vi "GM-UV-PAM.vi"() -> ()   [LabVIEW 2017]
uses:
  AlazarTech/ATS-VI/6.3.0/ATS_ctl/ATS_DMA_Channel.ctl
  <vilib>/userdefined/High Color/nirio_resource_hc.ctl
  <vilib>/FPGAPlugInAG/myRIO-1900/niLvFpga_Open_myRIO-1900.vi
  <vilib>/FPGAPlugInAG/myRIO-1900/niLvFpga_Reset_myRIO-1900.vi
  <vilib>/rvi/interface/common/niFpgaWaitOnOcc.vi
  <vilib>/Utility/error.llb/Error Cluster From Error Code.vi
  <vilib>/rvi/errors/niLvFpgaAdjustHostInterfaceError.vi
  <vilib>/FPGAPlugInAG/myRIO-1900/niLvFpga_Run_myRIO-1900.vi
  <vilib>/FPGAPlugInAG/myRIO-1900/niLvFpga_Close_myRIO-1900.vi
  <vilib>/rvi/interface/nirviOpenFPGA/nirviOpenFPGA.xnode
  FPGA Bitfiles/singlechannelMEM_FPGATarget2_MEMSMyRIO(FPGA)_jCEcXuE4l5k.lvbitx
  MEMS_MyRIO(FPGA).vi
  <vilib>/rvi/interface/nirviMethod/nirviMethod.xnode
  <vilib>/rvi/interface/nirviReadWriteControl/nirviReadWriteControl.xnode
  <vilib>/rvi/interface/nirviCloseFPGA/nirviCloseFPGA.xnode
  <vilib>/Analysis/NI_AALPro.lvlib
  <vilib>/rvi/errors/niLvFpgaMergeErrorWithErrorCode.vi
  NiFpgaLv.dll
  <vilib>/FPGAPlugInAG/myRIO-1900/niLvFpga_ConfigureFifo_myRIO-1900.vi
  <vilib>/FPGAPlugInAG/myRIO-1900/niLvFpga_WriteFifo_myRIO-1900.vi
panel:
  out "s? t:f":u16[](array[numeric])
  out "Pulses":u8[](array[numeric])
  out "Pulsesb":u8[](array[numeric])
  out "Timesperdx":i16
  in  "Savemap":bool
  in  "Calc MAP":bool
  in  "3D scan #":dbl=80.0
  out "B-scan #":u32=100
  in  "B-scan Rate":dbl=100.0 min=0.1 max=1000.0 step=0.1 format="%#_4g"
  in  "En":bool=TRUE
  in  "Mode":enum32{"Continuous", "Discrete"}(radio)
  in  "Step Size":dbl=16.0
  in  "Range (V) 2":sgl=2.0 format="%0.2f"
  in  "Offset(V)":dbl
  in  "Mirror PAM":enum32{"Main", "Others"}(tab)
  out "B-Scan 2":u16[][](graph)
  in  "pd delay":i16
  out "Laser/xn/dx should be an integer and not 1":string
  in  "Big_data":bool=TRUE
  in  "Zdiv":i8=2
  out "String 2":string="better<2^32"
  out "String":string="better<2000"
  out "Motorfreq_hz= Laserfre*dy/GMnum":dbl
  out "Stop_dispaly":bool
  in  "catbscan":i16=2
  in  "Laser Rep Rate":u32=10000 max=300000
  in  "Channel":T1
  in  "file path":path=path "G:/LXF/UV-PAM/test/test.dat"
  out "B-scan saved":i32=1600
  out "B-Scan":u16[][](graph)
  in  "Offset (V)":dbl format="%0.3f"
  in  "Range (V)":dbl=0.015 format="%0.3f"
  in  "Phase0(deg)":dbl format="%0.2f"
  in  "Trig. Delay (us)":sgl=4.3
  in  "Pt per A-line":i32=256
  in  "Rate":enum16{"500M", "250M", "125M"}(ring)
  in  "showmap":bool=TRUE
  in  "A/B-line show":bool=TRUE
  out "Alines":i32=320
  in  "Ele_Ini_Dir":bool=TRUE caption="Motor"
  out "Laser fired":i32=512000
  in  "zdir":bool
  in  "dy":i32=2 min=1 max=4
  in  "yn":i32=1000
  in  "kz":dbl=1.0
  in  "dx":i32=128
  in  "xEn":bool=TRUE
  in  "GMnum":i16=10
  in  "yEn":bool=TRUE
  in  "stop 2":bool
  in  "xn":i32=1000
  out "Waveform Graph":u16[][](graph)
  in  "ChA_Range":u32(ring)=5 items=["40 mV"=2, "100 mV"=5, "200 mV"=6, "400 mV"=7, "1 V"=10, "2 V"=11, "4 V"=12]
  in  "Triger Source":T2(ring)=enum."External"
  in  "Range Ch2":u32(ring)=3 items=["40mV", "100mV", "200mV", "400mV", "1 V", "2 V", "4 V"]
  in  "Trig Slope":enum32{"Positive", "Negative"}(ring)
  in  "Trig Level":u32=144
  out "C-Scan Ticks":dbl=300000.0
  out "Ch1 Pt":i32=384000
  out "DAQ Trig #":i32=3000
  out "Aline Stop #":i32=24000000
  out "DataQueue":refnum<queue>
  in  "signal type":T3(ring)=enum."triangle"
  out "Galvo Mirror Traj":i16[](graph)=[0, 0, 0, 1, 1, 1, 1, 2, 2, 2, 2, 2, 3, 3, 3, 3, 3, 4, 4, 4, 4, 5, 5, 5, 5, 5, 6, 6, 6, 6, 6, 7, 7, 7, 7, 7, 8, 8, 8, 8, 9, 9, 9, 9, 9, 10, 10, 10, 10, 10, 11, 11, 11, 11, 12, 12, 12, 12, 12, 13, 13, 13, 13, 13, 14, 14, 14, 14, 15, 15, 15, 15, 15, 16, 16, 16, 16, 16, 17, 17, 17, 17, 17, 18, 18, 18, 18, 19, 19, 19, 19, 19, 20, 20, 20, 20, 20, 21, 21, 21, 21, 21, 22, 22, 22, 22, 23, 23, 23, 23, 23, 24, 24, 24, 24, 24, 25, 25, 25, 25, 25, 26, 26, 26, 26, 27, 27, 27, 27, 27, 28, 28, 28, 28, 28, 29, 29, 29, 29, 29, 30, 30, 30, 30, 30, 31, 31, 31, 31, 31, 32, 32, 32, 32, 32, 33, 33, 33, 33, 33, 34, 34, 34, 34, 34, 35, 35, 35, 35, 35, 36, 36, 36, 36, 36, 37, 37, 37, 37, 37, 38, 38, 38, 38, 38, 39, 39, 39, 39, 39, 40, 40, 40, 40, 40, 41, 41, 41, 41, 41, 42, 42, 42, 42, 42, 43, 43, 43, 43, 43, 44, 44, 44, 44, 44, 45, 45, 45, 45, 45, 46, 46, 46, 46, 46, 46, 47, 47, 47, 47, 47, 48, 48, 48, 48, 48, 49, 49, 49, 49, 49, 50, 50, 50, 50, 50, 50, 51, 51, 51, 51, 51, 52, 52, 52, 52, 52, 52, 53, 53, 53, 53, 53, 54, 54, 54, 54, 54, 55, 55, 55, 55, 55, 55, 56, 56, 56, 56, 56, 56, 57, 57, 57, 57, 57, 58, 58, 58, 58, 58, 58, 59, 59, 59, 59, 59, 59, 60, 60, 60, 60, 60, 61, 61, 61, 61, 61, 61, 62, 62, 62, 62, 62, 62, 63, 63, 63, 63, 63, 63, 64, 64, 64, 64, 64, 64, 65, 65, 65, 65, 65, 65, 66, 66, 66, 66, 66, 66, 67, 67, 67, 67, 67, 67, 68, 68, 68, 68, 68, 68, 69, 69, 69, 69, 69, 69, 69, 70, 70, 70, 70, 70, 70, 71, 71, 71, 71, 71, 71, 71, 72, 72, 72, 72, 72, 72, 73, 73, 73, 73, 73, 73, 73, 74, 74, 74, 74, 74, 74, 74, 75, 75, 75, 75, 75, 75, 76, 76, 76, 76, 76, 76, 76, 77, 77, 77, 77, 77, 77, 77, 78, 78, 78, 78, 78, 78, 78, 78, 79, 79, 79, 79, 79, 79, 79, 80, 80, 80, 80, 80, 80, 80, 81, 81, 81, 81, 81, 81, 81, 81, 82, 82, 82, 82, 82, 82, 82, 82, 83, 83, 83, 83, 83, 83, 83, 83, 84, 84, 84, 84, 84, 84, 84, 84, 85, 85, 85, 85, 85, 85, 85, 85, 86, 86, 86, 86, 86, 86, 86, 86, 86, 87, 87, 87, 87, 87, 87, 87, 87, 87, 88, 88, 88, 88, 88, 88, 88, 88, 88, 89, 89, 89, 89, 89, 89, 89, 89, 89, 90, 90, 90, 90, 90, 90, 90, 90, 90, 90, 91, 91, 91, 91, 91, 91, 91, 91, 91, 91, 92, 92, 92, 92, 92, 92, 92, 92, 92, 92, 92, 93, 93, 93, 93, 93, 93, 93, 93, 93, 93, 93, 94, 94, 94, 94, 94, 94, 94, 94, 94, 94, 94, 94, 95, 95, 95, 95, 95, 95, 95, 95, 95, 95, 95, 95, 96, 96, 96, 96, 96, 96, 96, 96, 96, 96, 96, 96, 96, 96, 97, 97, 97, 97, 97, 97, 97, 97, 97, 97, 97, 97, 97, 97, 98, 98, 98, 98, 98, 98, 98, 98, 98, 98, 98, 98, 98, 98, 98, 98, 99, 99, 99, 99, 99, 99, 99, 99, 99, 99, 99, 99, 99, 99, 99, 99, 99, 99, 99, 100, 100, 100, 100, 100, 100, 100, 100, 100, 100, 100, 100, 100, 100, 100, 100, 100, 100, 100, 100, 100, 101, 101, 101, 101, 101, 101, 101, 101, 101, 101, 101, 101, 101, 101, 101, 101, 101, 101, 101, 101, 101, 101, 101, 101, 101, 101, 101, 101, 101, 102, 102, 102, 102, 102, 102, 102, 102, 102, 102, 102, 102, 102, 102, 102, 102, 102, 102, 102, 102, 102, 102, 102, 102, 102, 102, 102, 102, 102, 102, 102, 102, 102, 102, 102, 102, 102, 102, 102, 102, 102, 102, 102, 102, 102, 102, 102, 102, 102, 102, 102, 102, 102, 102, 102, 102, 102, 102, 102, 102, 102, 102, 102, 102, 102, 102, 102, 102, 102, 102, 102, 102, 102, 102, 102, 102, 102, 102, 102, 102, 102, 102, 102, 102, 102, 102, 102, 102, 102, 102, 102, 102, 102, 102, 102, 102, 102, 102, 102, 102, 102, 102, 102, 102, 102, 102, 102, 102, 102, 102, 102, 102, 102, 102, 102, 102, 102, 102, 102, 102, 102, 102, 102, 102, 102, 102, 102, 101, 101, 101, 101, 101, 101, 101, 101, 101, 101, 101, 101, 101, 101, 101, 101, 101, 101, 101, 101, 101, 101, 101, 101, 101, 101, 101, 101, 101, 100, 100, 100, 100, 100, 100, 100, 100, 100, 100, 100, 100, 100, 100, 100, 100, 100, 100, 100, 100, 100, 99, 99, 99, 99, 99, 99, 99, 99, 99, 99, 99, 99, 99, 99, 99, 99, 99, 99, 99, 98, 98, 98, 98, 98, 98, 98, 98, 98, 98, 98, 98, 98, 98, 98, 98, 97, 97, 97, 97, 97, 97, 97, 97, 97, 97, 97, 97, 97, 97, 96, 96, 96, 96, 96, 96, 96, 96, 96, 96, 96, 96, 96, 96, 95, 95, 95, 95, 95, 95, 95, 95, 95, 95, 95, 95, 94, 94, 94, 94, 94, 94, 94, 94, 94, 94, 94, 94, 93, 93, 93, 93, 93, 93, 93, 93, 93, 93, 93, 92, 92, 92, 92, 92, 92, 92, 92, 92, 92, 92, 91, 91, 91, 91, 91, 91, 91, 91, 91, 91, 90, 90, 90, 90, 90, 90, 90, 90, 90, 90, 89, 89, 89, 89, 89, 89, 89, 89, 89, 88, 88, 88, 88, 88, 88, 88, 88, 88, 87, 87, 87, 87, 87, 87, 87, 87, 87, 86, 86, 86, 86, 86, 86, 86, 86, 86, 85, 85, 85, 85, 85, 85, 85, 85, 84, 84, 84, 84, 84, 84, 84, 84, 83, 83, 83, 83, 83, 83, 83, 83, 82, 82, 82, 82, 82, 82, 82, 82, 81, 81, 81, 81, 81, 81, 81, 81, 80, 80, 80, 80, 80, 80, 80, 79, 79, 79, 79, 79, 79, 79, 78, 78, 78, 78, 78, 78, 78, 78, 77, 77, 77, 77, 77, 77, 77, 76, 76, 76, 76, 76, 76, 76, 75, 75, 75, 75, 75, 75, 74, 74, 74, 74, 74, 74, 74, 73, 73, 73, 73, 73, 73, 73, 72, 72, 72, 72, 72, 72, 71, 71, 71, 71, 71, 71, 71, 70, 70, 70, 70, 70, 70, 69, 69, 69, 69, 69, 69, 69, 68, 68, 68, 68, 68, 68, 67, 67, 67, 67, 67, 67, 66, 66, 66, 66, 66, 66, 65, 65, 65, 65, 65, 65, 64, 64, 64, 64, 64, 64, 63, 63, 63, 63, 63, 63, 62, 62, 62, 62, 62, 62, 61, 61, 61, 61, 61, 61, 60, 60, 60, 60, 60, 59, 59, 59, 59, 59, 59, 58, 58, 58, 58, 58, 58, 57, 57, 57, 57, 57, 56, 56, 56, 56, 56, 56, 55, 55, 55, 55, 55, 55, 54, 54, 54, 54, 54, 53, 53, 53, 53, 53, 52, 52, 52, 52, 52, 52, 51, 51, 51, 51, 51, 50, 50, 50, 50, 50, 50, 49, 49, 49, 49, 49, 48, 48, 48, 48, 48, 47, 47, 47, 47, 47, 46, 46, 46, 46, 46, 46, 45, 45, 45, 45, 45, 44, 44, 44, 44, 44, 43, 43, 43, 43, 43, 42, 42, 42, 42, 42, 41, 41, 41, 41, 41, 40, 40, 40, 40, 40, 39, 39, 39, 39, 39, 38, 38, 38, 38, 38, 37, 37, 37, 37, 37, 36, 36, 36, 36, 36, 35, 35, 35, 35, 35, 34, 34, 34, 34, 34, 33, 33, 33, 33, 33, 32, 32, 32, 32, 32, 31, 31, 31, 31, 31, 30, 30, 30, 30, 30, 29, 29, 29, 29, 29, 28, 28, 28, 28, 28, 27, 27, 27, 27, 27, 26, 26, 26, 26, 25, 25, 25, 25, 25, 24, 24, 24, 24, 24, 23, 23, 23, 23, 23, 22, 22, 22, 22, 21, 21, 21, 21, 21, 20, 20, 20, 20, 20, 19, 19, 19, 19, 19, 18, 18, 18, 18, 17, 17, 17, 17, 17, 16, 16, 16, 16, 16, 15, 15, 15, 15, 15, 14, 14, 14, 14, 13, 13, 13, 13, 13, 12, 12, 12, 12, 12, 11, 11, 11, 11, 10, 10, 10, 10, 10, 9, 9, 9, 9, 9, 8, 8, 8, 8, 7, 7, 7, 7, 7, 6, 6, 6, 6, 6, 5, 5, 5, 5, 5, 4, 4, 4, 4, 3, 3, 3, 3, 3, 2, 2, 2, 2, 2, 1, 1, 1, 1, 0, 0, 0, 0, 0, -1, -1, -1, -1, -2, -2, -2, -2, -2, -3, -3, -3, -3, -3, -4, -4, -4, -4, -5, -5, -5, -5, -5, -6, -6, -6, -6, -6, -7, -7, -7, -7, -7, -8, -8, -8, -8, -9, -9, -9, -9, -9, -10, -10, -10, -10, -10, -11, -11, -11, -11, -12, -12, -12, -12, -12, -13, -13, -13, -13, -13, -14, -14, -14, -14, -15, -15, -15, -15, -15, -16, -16, -16, -16, -16, -17, -17, -17, -17, -17, -18, -18, -18, -18, -19, -19, -19, -19, -19, -20, -20, -20, -20, -20, -21, -21, -21, -21, -21, -22, -22, -22, -22, -23, -23, -23, -23, -23, -24, -24, -24, -24, -24, -25, -25, -25, -25, -25, -26, -26, -26, -26, -27, -27, -27, -27, -27, -28, -28, -28, -28, -28, -29, -29, -29, -29, -29, -30, -30, -30, -30, -30, -31, -31, -31, -31, -31, -32, -32, -32, -32, -32, -33, -33, -33, -33, -33, -34, -34, -34, -34, -34, -35, -35, -35, -35, -35, -36, -36, -36, -36, -36, -37, -37, -37, -37, -37, -38, -38, -38, -38, -38, -39, -39, -39, -39, -39, -40, -40, -40, -40, -40, -41, -41, -41, -41, -41, -42, -42, -42, -42, -42, -43, -43, -43, -43, -43, -44, -44, -44, -44, -44, -45, -45, -45, -45, -45, -46, -46, -46, -46, -46, -46, -47, -47, -47, -47, -47, -48, -48, -48, -48, -48, -49, -49, -49, -49, -49, -50, -50, -50, -50, -50, -50, -51, -51, -51, -51, -51, -52, -52, -52, -52, -52, -52, -53, -53, -53, -53, -53, -54, -54, -54, -54, -54, -55, -55, -55, -55, -55, -55, -56, -56, -56, -56, -56, -56, -57, -57, -57, -57, -57, -58, -58, -58, -58, -58, -58, -59, -59, -59, -59, -59, -59, -60, -60, -60, -60, -60, -61, -61, -61, -61, -61, -61, -62, -62, -62, -62, -62, -62, -63, -63, -63, -63, -63, -63, -64, -64, -64, -64, -64, -64, -65, -65, -65, -65, -65, -65, -66, -66, -66, -66, -66, -66, -67, -67, -67, -67, -67, -67, -68, -68, -68, -68, -68, -68, -69, -69, -69, -69, -69, -69, -69, -70, -70, -70, -70, -70, -70, -71, -71, -71, -71, -71, -71, -71, -72, -72, -72, -72, -72, -72, -73, -73, -73, -73, -73, -73, -73, -74, -74, -74, -74, -74, -74, -74, -75, -75, -75, -75, -75, -75, -76, -76, -76, -76, -76, -76, -76, -77, -77, -77, -77, -77, -77, -77, -78, -78, -78, -78, -78, -78, -78, -78, -79, -79, -79, -79, -79, -79, -79, -80, -80, -80, -80, -80, -80, -80, -81, -81, -81, -81, -81, -81, -81, -81, -82, -82, -82, -82, -82, -82, -82, -82, -83, -83, -83, -83, -83, -83, -83, -83, -84, -84, -84, -84, -84, -84, -84, -84, -85, -85, -85, -85, -85, -85, -85, -85, -86, -86, -86, -86, -86, -86, -86, -86, -86, -87, -87, -87, -87, -87, -87, -87, -87, -87, -88, -88, -88, -88, -88, -88, -88, -88, -88, -89, -89, -89, -89, -89, -89, -89, -89, -89, -90, -90, -90, -90, -90, -90, -90, -90, -90, -90, -91, -91, -91, -91, -91, -91, -91, -91, -91, -91, -92, -92, -92, -92, -92, -92, -92, -92, -92, -92, -92, -93, -93, -93, -93, -93, -93, -93, -93, -93, -93, -93, -94, -94, -94, -94, -94, -94, -94, -94, -94, -94, -94, -94, -95, -95, -95, -95, -95, -95, -95, -95, -95, -95, -95, -95, -96, -96, -96, -96, -96, -96, -96, -96, -96, -96, -96, -96, -96, -96, -97, -97, -97, -97, -97, -97, -97, -97, -97, -97, -97, -97, -97, -97, -98, -98, -98, -98, -98, -98, -98, -98, -98, -98, -98, -98, -98, -98, -98, -98, -99, -99, -99, -99, -99, -99, -99, -99, -99, -99, -99, -99, -99, -99, -99, -99, -99, -99, -99, -100, -100, -100, -100, -100, -100, -100, -100, -100, -100, -100, -100, -100, -100, -100, -100, -100, -100, -100, -100, -100, -101, -101, -101, -101, -101, -101, -101, -101, -101, -101, -101, -101, -101, -101, -101, -101, -101, -101, -101, -101, -101, -101, -101, -101, -101, -101, -101, -101, -101, -102, -102, -102, -102, -102, -102, -102, -102, -102, -102, -102, -102, -102, -102, -102, -102, -102, -102, -102, -102, -102, -102, -102, -102, -102, -102, -102, -102, -102, -102, -102, -102, -102, -102, -102, -102, -102, -102, -102, -102, -102, -102, -102, -102, -102, -102, -102, -102, -102, -102, -102, -102, -102, -102, -102, -102, -102, -102, -102, -102, -102, -102, -102, -102, -102, -102, -102, -102, -102, -102, -102, -102, -102, -102, -102, -102, -102, -102, -102, -102, -102, -102, -102, -102, -102, -102, -102, -102, -102, -102, -102, -102, -102, -102, -102, -102, -102, -102, -102, -102, -102, -102, -102, -102, -102, -102, -102, -102, -102, -102, -102, -102, -102, -102, -102, -102, -102, -102, -102, -102, -102, -102, -102, -102, -102, -102, -102, -101, -101, -101, -101, -101, -101, -101, -101, -101, -101, -101, -101, -101, -101, -101, -101, -101, -101, -101, -101, -101, -101, -101, -101, -101, -101, -101, -101, -101, -100, -100, -100, -100, -100, -100, -100, -100, -100, -100, -100, -100, -100, -100, -100, -100, -100, -100, -100, -100, -100, -99, -99, -99, -99, -99, -99, -99, -99, -99, -99, -99, -99, -99, -99, -99, -99, -99, -99, -99, -98, -98, -98, -98, -98, -98, -98, -98, -98, -98, -98, -98, -98, -98, -98, -98, -97, -97, -97, -97, -97, -97, -97, -97, -97, -97, -97, -97, -97, -97, -96, -96, -96, -96, -96, -96, -96, -96, -96, -96, -96, -96, -96, -96, -95, -95, -95, -95, -95, -95, -95, -95, -95, -95, -95, -95, -94, -94, -94, -94, -94, -94, -94, -94, -94, -94, -94, -94, -93, -93, -93, -93, -93, -93, -93, -93, -93, -93, -93, -92, -92, -92, -92, -92, -92, -92, -92, -92, -92, -92, -91, -91, -91, -91, -91, -91, -91, -91, -91, -91, -90, -90, -90, -90, -90, -90, -90, -90, -90, -90, -89, -89, -89, -89, -89, -89, -89, -89, -89, -88, -88, -88, -88, -88, -88, -88, -88, -88, -87, -87, -87, -87, -87, -87, -87, -87, -87, -86, -86, -86, -86, -86, -86, -86, -86, -86, -85, -85, -85, -85, -85, -85, -85, -85, -84, -84, -84, -84, -84, -84, -84, -84, -83, -83, -83, -83, -83, -83, -83, -83, -82, -82, -82, -82, -82, -82, -82, -82, -81, -81, -81, -81, -81, -81, -81, -81, -80, -80, -80, -80, -80, -80, -80, -79, -79, -79, -79, -79, -79, -79, -78, -78, -78, -78, -78, -78, -78, -78, -77, -77, -77, -77, -77, -77, -77, -76, -76, -76, -76, -76, -76, -76, -75, -75, -75, -75, -75, -75, -74, -74, -74, -74, -74, -74, -74, -73, -73, -73, -73, -73, -73, -73, -72, -72, -72, -72, -72, -72, -71, -71, -71, -71, -71, -71, -71, -70, -70, -70, -70, -70, -70, -69, -69, -69, -69, -69, -69, -69, -68, -68, -68, -68, -68, -68, -67, -67, -67, -67, -67, -67, -66, -66, -66, -66, -66, -66, -65, -65, -65, -65, -65, -65, -64, -64, -64, -64, -64, -64, -63, -63, -63, -63, -63, -63, -62, -62, -62, -62, -62, -62, -61, -61, -61, -61, -61, -61, -60, -60, -60, -60, -60, -59, -59, -59, -59, -59, -59, -58, -58, -58, -58, -58, -58, -57, -57, -57, -57, -57, -56, -56, -56, -56, -56, -56, -55, -55, -55, -55, -55, -55, -54, -54, -54, -54, -54, -53, -53, -53, -53, -53, -52, -52, -52, -52, -52, -52, -51, -51, -51, -51, -51, -50, -50, -50, -50, -50, -50, -49, -49, -49, -49, -49, -48, -48, -48, -48, -48, -47, -47, -47, -47, -47, -46, -46, -46, -46, -46, -46, -45, -45, -45, -45, -45, -44, -44, -44, -44, -44, -43, -43, -43, -43, -43, -42, -42, -42, -42, -42, -41, -41, -41, -41, -41, -40, -40, -40, -40, -40, -39, -39, -39, -39, -39, -38, -38, -38, -38, -38, -37, -37, -37, -37, -37, -36, -36, -36, -36, -36, -35, -35, -35, -35, -35, -34, -34, -34, -34, -34, -33, -33, -33, -33, -33, -32, -32, -32, -32, -32, -31, -31, -31, -31, -31, -30, -30, -30, -30, -30, -29, -29, -29, -29, -29, -28, -28, -28, -28, -28, -27, -27, -27, -27, -27, -26, -26, -26, -26, -25, -25, -25, -25, -25, -24, -24, -24, -24, -24, -23, -23, -23, -23, -23, -22, -22, -22, -22, -21, -21, -21, -21, -21, -20, -20, -20, -20, -20, -19, -19, -19, -19, -19, -18, -18, -18, -18, -17, -17, -17, -17, -17, -16, -16, -16, -16, -16, -15, -15, -15, -15, -15, -14, -14, -14, -14, -13, -13, -13, -13, -13, -12, -12, -12, -12, -12, -11, -11, -11, -11, -10, -10, -10, -10, -10, -9, -9, -9, -9, -9, -8, -8, -8, -8, -7, -7, -7, -7, -7, -6, -6, -6, -6, -6, -5, -5, -5, -5, -5, -4, -4, -4, -4, -3, -3, -3, -3, -3, -2, -2, -2, -2, -2, -1, -1, -1, -1, 0, 0]
  in  "save_rate":u32=5
  in  "DO_rate_tick":u32=2000
  in  "Laserupdateus":u32=2000
  out "Graph":u16[][](graph)
  out "Trigger pulse graph 2":digitalwaveform(graph)={"t0"=timestamp(0 s since 1904-01-01), "dt"=0.025, "Y"={"transitions"=[], "data"=array1242x4[4968 elements]}}
  in  "Dual Wave":bool=TRUE
  in  "Split":i32=28
  out "MAP":u16[][](graph)
  out "file_ref":refnum<file>
  # "Scan"
  # "Step motor"
  # "Y Mirror"
  # "Max Rep rate 310 kHz"
  # "AD"
  # "Galvo Mirror"
  # "DAQ"
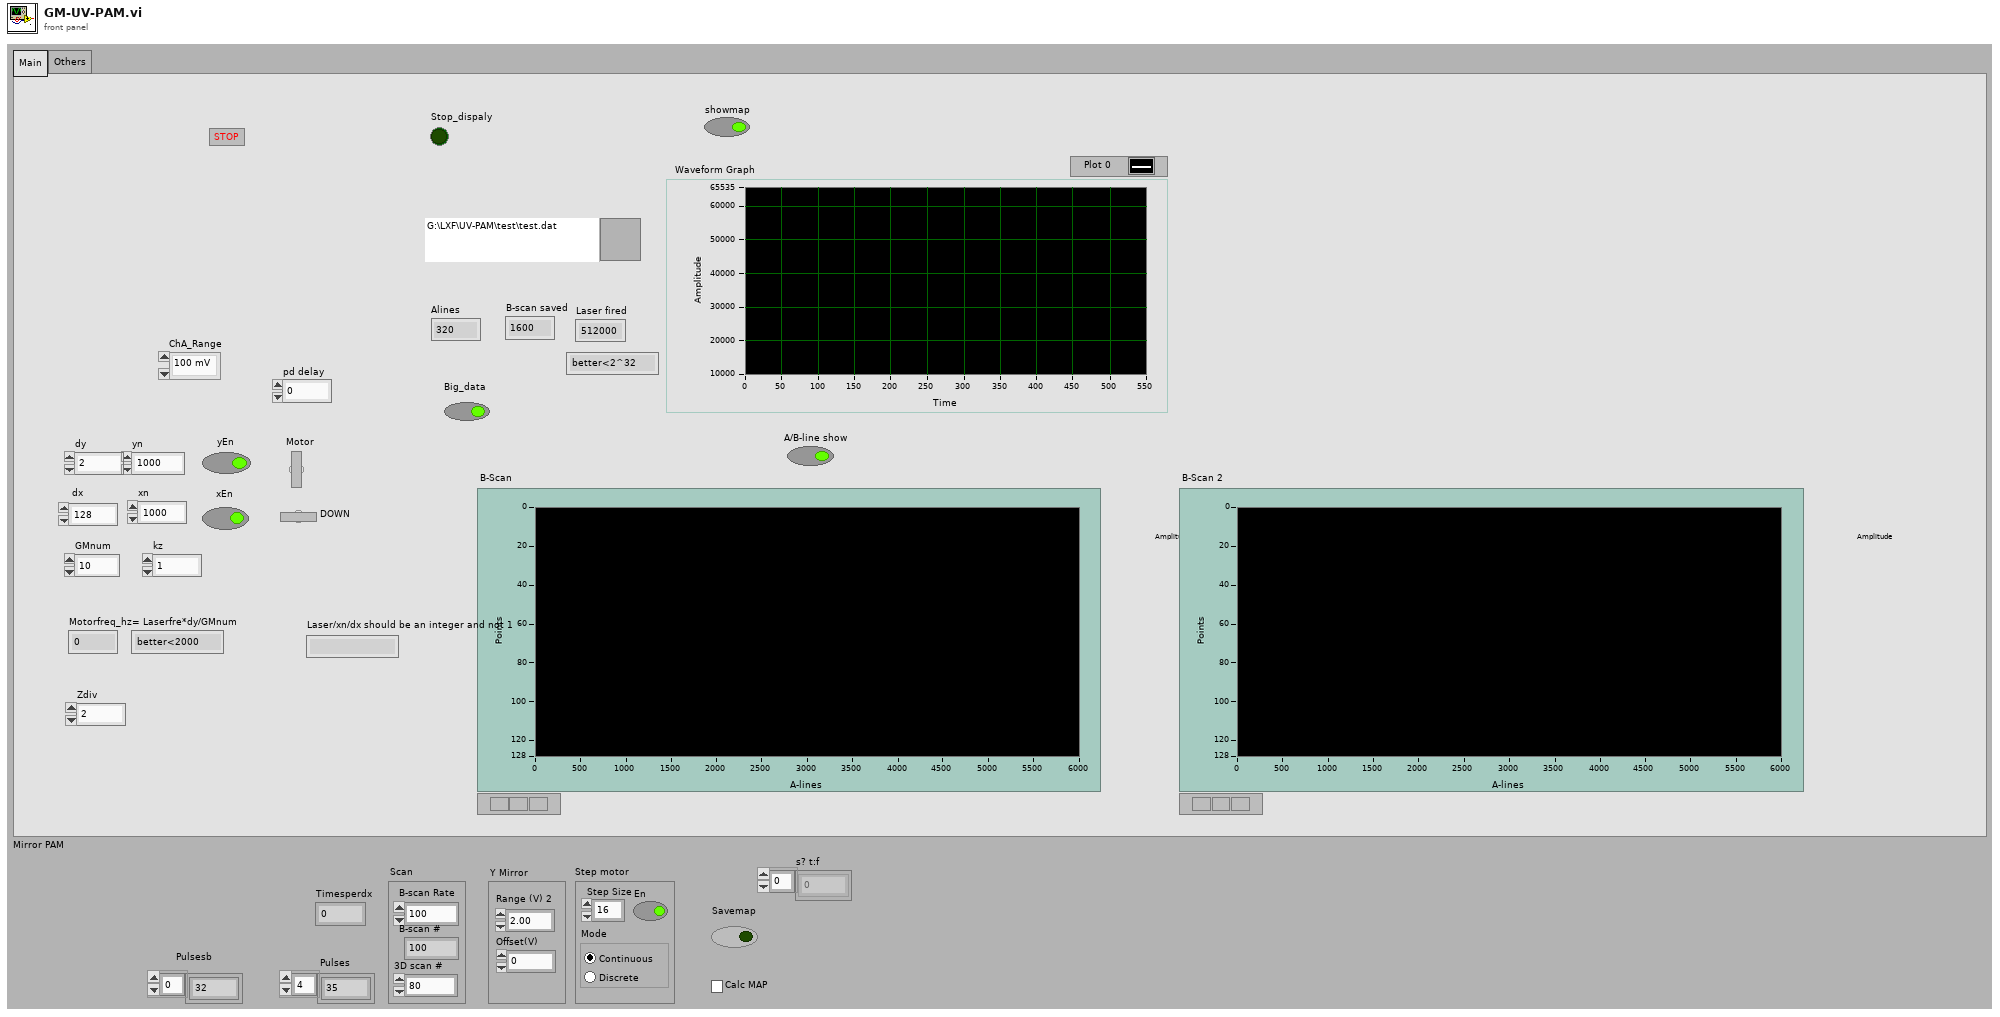
[diagram p1: front panel]
types:
  T1 = typedef "ATS_DMA_Channel.ctl" = enum16{"Channel_A", "Channel_B", "A & B"}
  T2 = enum32{"Chan_A", "Chan_B", "External", "Disable"}
  T3 = enum16{"sine", "cosine", "triangle", "square", "sawtooth", "increasing ramp", "decreasing ramp"}
  T4 = enum16{"open", "replace", "create", "open or create", "replace or create", "replace or create with confirmation"}
  T5 = enum16{"big-endian, network order", "native, host order", "little-endian"}
  T6 = typedef "nirio_resource_hc.ctl" = tag
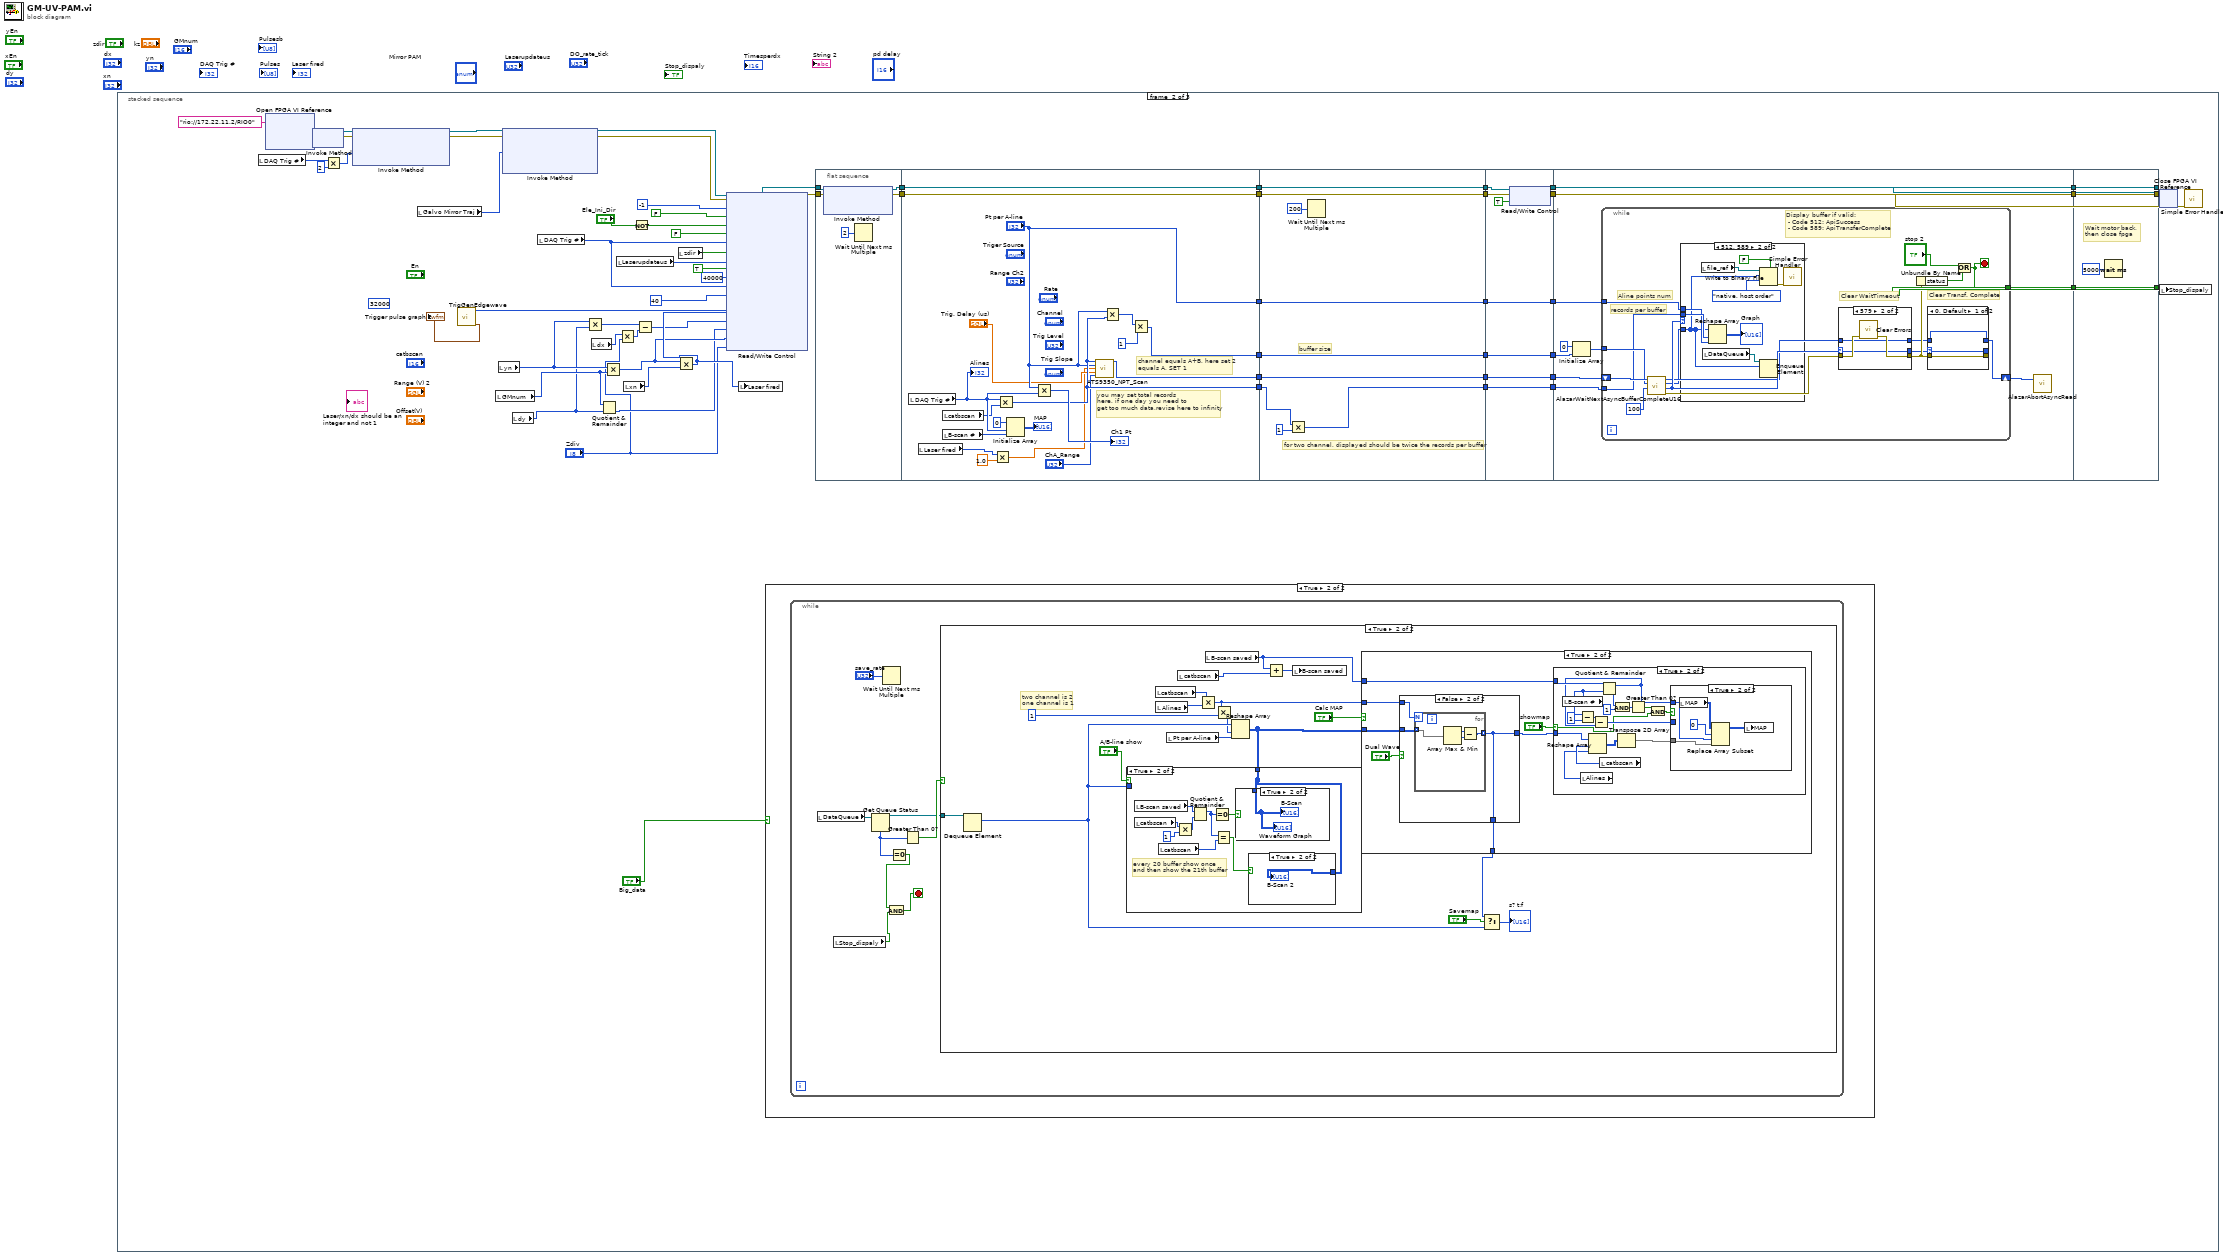
[diagram p0: block diagram]
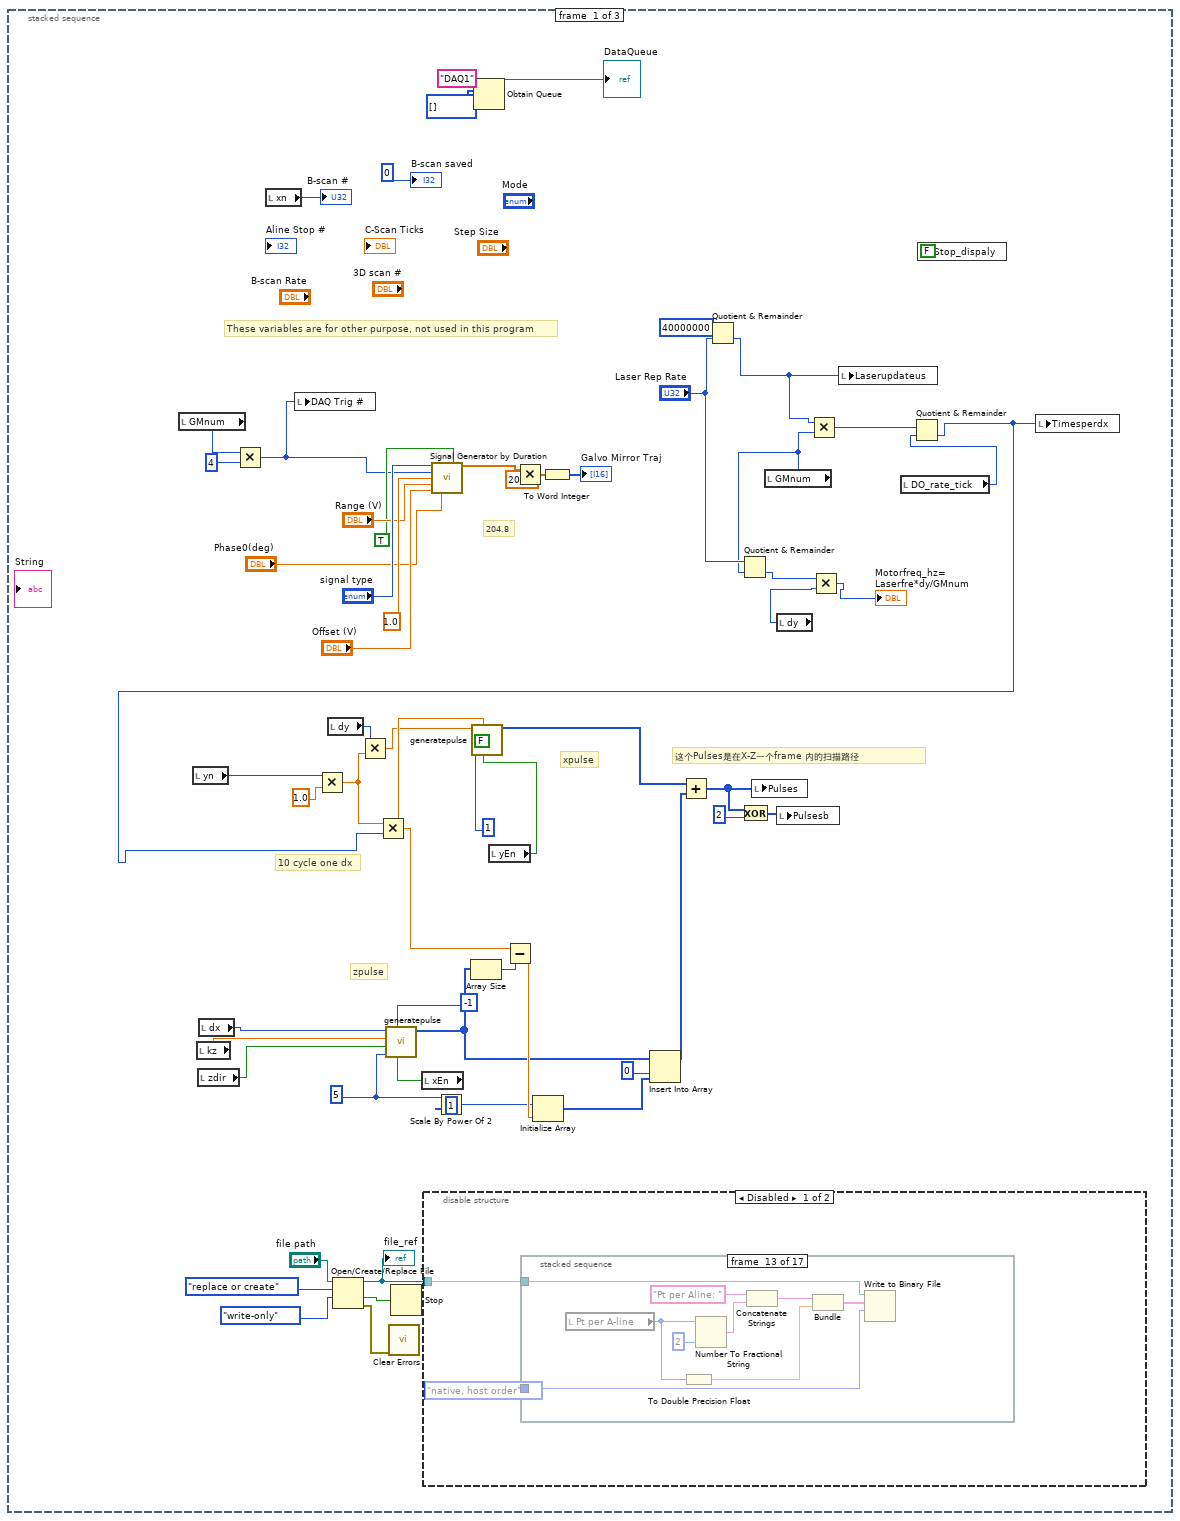
[diagram p2: hidden frame]
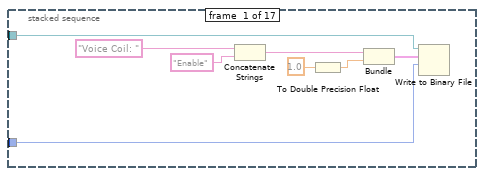
[diagram p3: hidden frame]
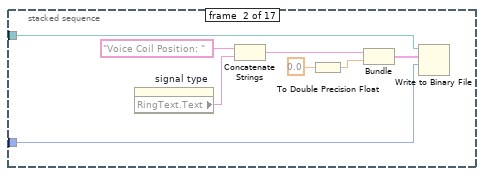
[diagram p4: hidden frame]
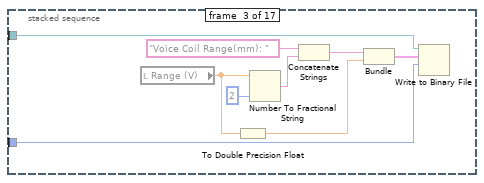
[diagram p5: hidden frame]
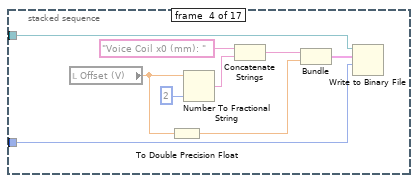
[diagram p6: hidden frame]
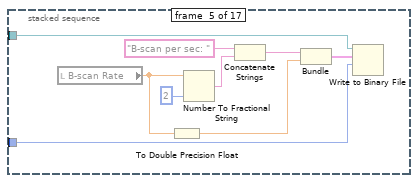
[diagram p7: hidden frame]
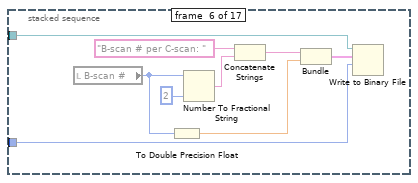
[diagram p8: hidden frame]
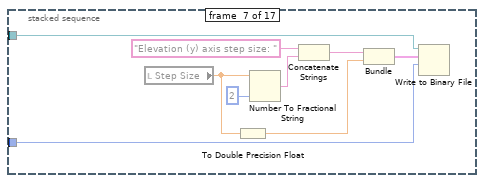
[diagram p9: hidden frame]
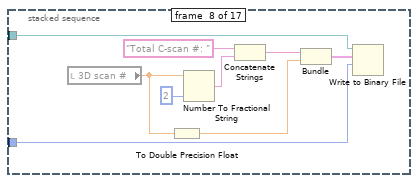
[diagram p10: hidden frame]
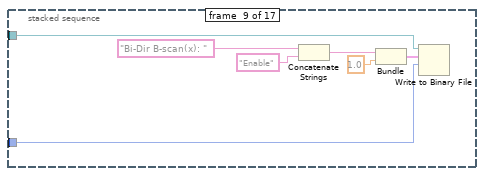
[diagram p11: hidden frame]
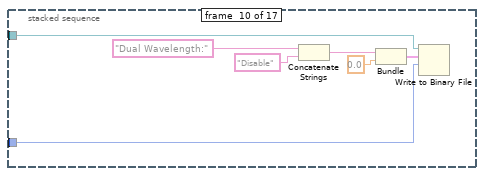
[diagram p12: hidden frame]
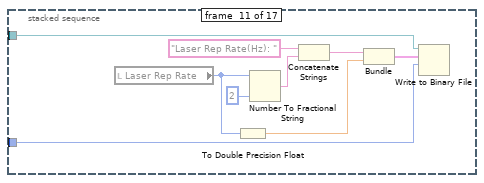
[diagram p13: hidden frame]
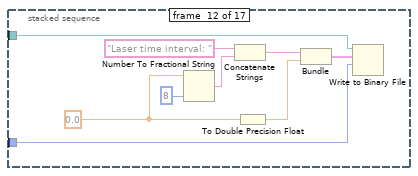
[diagram p14: hidden frame]
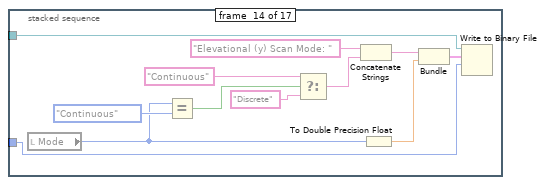
[diagram p15: hidden frame]
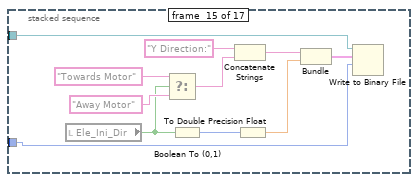
[diagram p16: hidden frame]
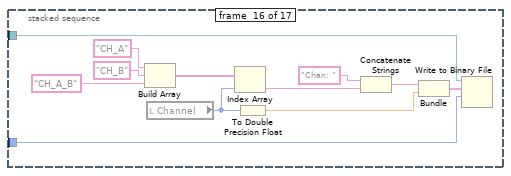
[diagram p17: hidden frame]
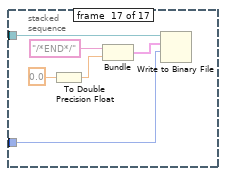
[diagram p18: hidden frame]
diagram:
  n1 = stacked-sequence {
    frame #0 {
      w18 = u8 5 ("bit")
      # "These variables are for other purpose, not used in this program"
      # "10 cycle one dx"
      # "这个Pulses是在X-Z一个frame 内的扫描路径"
      # "zpulse"
      # "xpulse"
      # "204.8"
      n2 = local read "GMnum"() -> (w16:i16)
      n3 = local read "yn"() -> (w40:i32)
      n4 = local read "kz"() -> (w24:dbl)
      n5 = local read "zdir"() -> (w23:bool)
      n6 = local read "dx"() -> (w25:i32)
      n7 = Multiply(x=w16, y=i16 4) -> (x*y=w14:i16)
      n8 = local read "xn"() -> (→"B-scan #":i32)
      n9 = local write "DAQ Trig #"(w14) -> ()
      n10 = Multiply(x=w40, y=1.0) -> (x*y=w42:dbl)
      n11 = local read "dy"() -> (w41:i32)
      n12 = Open/Create/Replace File(file path (use dialog)="file path", operation (0:open)=T4."replace or create", access (0:read/write)=enum16{"read/write", "read-only", "write-only"}."write-only") -> (refnum out=w48:refnum<file>, cancelled=w47:bool, error out=w46:errorcluster)  [unwired: 1 in, 2 out]
      "file_ref" <- w48
      n13 = Multiply(x=w41, y=w42) -> (x*y=w30:dbl)
      n14 = call <vilib>:"Clear Errors.vi"("error in (no error)"=w46) -> ()  [unwired: 5 in, 2 out]
      n15 = Stop(stop? (T)=w47) -> ()
      n16 = local read "xEn"() -> (w22:bool)
      n17 = call "generatepulse.vi"("en"=w22, "samples"=-1, "bit"=w18, "dir"=w23, "kx"=w24, "xn"=w25) -> ("pulsetrain"=w21:u8[])  [unwired: 5 in]
      n18 = disable-structure shown="Disabled" {
        disable-tunnel: w48 -> [w63 _]
        frame Disabled {
          n19 = stacked-sequence {
            tunnel: w63 -> [w71 w80 w89 w98 w104 w112 w123 w131 w141 w148 w154 w163 w171 w184 w194 w209 w215]
            tunnel: T5."native, host order" ("byte order (0:big-endian, network order)") -> [w72 w79 w88 w97 w103 w113 w122 w130 w140 w147 w153 w162 w172 w183 w193 w208 w216]
            frame #0 {
              n20 = Concatenate Strings("Voice Coil: " ("string"), "Enable") -> (w68:string)
              n21 = To Double Precision Float(number=1.0) -> (double precision float=w69:dbl)
              n22 = Bundle(w68, w69) -> (w67:cluster{string, dbl})  [unwired: 1 in]
              n23 = Write to Binary File(file (use dialog)=w71, data=w67, 9:w72) -> ()  [unwired: 3 in, 3 out]
            }
            frame #1 {
              n24 = property on="signal type" class="Enum (strict)"() -> ("RingText.Text"=w78:string)  [unwired: 2 in, 2 out]
              n25 = Concatenate Strings("Voice Coil Position: " ("string"), w78) -> (w74:string)
              n26 = To Double Precision Float(number=0.0) -> (double precision float=w76:dbl)
              n27 = Bundle(w74, w76) -> (w75:cluster{string, dbl})  [unwired: 1 in]
              n28 = Write to Binary File(file (use dialog)=w80, data=w75, 9:w79) -> ()  [unwired: 2 in, 4 out]
            }
            frame #2 {
              n29 = local read "Range (V)"() -> (w81:dbl)
              n30 = To Double Precision Float(number=w81) -> (double precision float=w84:dbl)
              n31 = Number To Fractional String(number=w81, precision (6)=i16 2) -> (F-format string=w86:string)  [unwired: 2 in]
              n32 = Concatenate Strings("Voice Coil Range(mm): " ("string"), w86) -> (w82:string)
              n33 = Bundle(w82, w84) -> (w83:cluster{string, dbl})  [unwired: 1 in]
              n34 = Write to Binary File(file (use dialog)=w89, data=w83, 9:w88) -> ()  [unwired: 2 in, 4 out]
            }
            frame #3 {
              n35 = local read "Offset (V)"() -> (w90:dbl)
              n36 = To Double Precision Float(number=w90) -> (double precision float=w93:dbl)
              n37 = Number To Fractional String(number=w90, precision (6)=i16 2) -> (F-format string=w95:string)  [unwired: 2 in]
              n38 = Concatenate Strings("Voice Coil x0 (mm): " ("string"), w95) -> (w91:string)
              n39 = Bundle(w91, w93) -> (w92:cluster{string, dbl})  [unwired: 1 in]
              n40 = Write to Binary File(file (use dialog)=w98, data=w92, 9:w97) -> ()  [unwired: 2 in, 4 out]
            }
            frame #4 {
              n41 = local read "B-scan Rate"() -> (w99:dbl)
              n42 = To Double Precision Float(number=w99) -> (double precision float=w102:dbl)
              n43 = Number To Fractional String(number=w99, precision (6)=i16 2) -> (F-format string=w106:string)  [unwired: 2 in]
              n44 = Concatenate Strings("B-scan per sec: " ("string"), w106) -> (w100:string)
              n45 = Bundle(w100, w102) -> (w101:cluster{string, dbl})  [unwired: 1 in]
              n46 = Write to Binary File(file (use dialog)=w104, data=w101, 9:w103) -> ()  [unwired: 2 in, 4 out]
            }
            frame #5 {
              n47 = local read "B-scan #"() -> (w108:u32)
              n48 = To Double Precision Float(number=w108) -> (double precision float=w111:dbl)
              n49 = Number To Fractional String(number=w108, precision (6)=i16 2) -> (F-format string=w115:string)  [unwired: 2 in]
              n50 = Concatenate Strings("B-scan # per C-scan: " ("string"), w115) -> (w109:string)
              n51 = Bundle(w109, w111) -> (w110:cluster{string, dbl})  [unwired: 1 in]
              n52 = Write to Binary File(file (use dialog)=w112, data=w110, 9:w113) -> ()  [unwired: 2 in, 4 out]
            }
            frame #6 {
              n53 = local read "Step Size"() -> (w117:dbl)
              n54 = To Double Precision Float(number=w117) -> (double precision float=w120:dbl)
              n55 = Number To Fractional String(number=w117, precision (6)=i16 2) -> (F-format string=w121:string)  [unwired: 2 in]
              n56 = Concatenate Strings("Elevation (y) axis step size: " ("string"), w121) -> (w118:string)
              n57 = Bundle(w118, w120) -> (w119:cluster{string, dbl})  [unwired: 1 in]
              n58 = Write to Binary File(file (use dialog)=w123, data=w119, 9:w122) -> ()  [unwired: 2 in, 4 out]
            }
            frame #7 {
              n59 = local read "3D scan #"() -> (w126:dbl)
              n60 = To Double Precision Float(number=w126) -> (double precision float=w129:dbl)
              n61 = Number To Fractional String(number=w126, precision (6)=i16 2) -> (F-format string=w133:string)  [unwired: 2 in]
              n62 = Concatenate Strings("Total C-scan #: " ("string"), w133) -> (w127:string)
              n63 = Bundle(w127, w129) -> (w128:cluster{string, dbl})  [unwired: 1 in]
              n64 = Write to Binary File(file (use dialog)=w131, data=w128, 9:w130) -> ()  [unwired: 2 in, 4 out]
            }
            frame #8 {
              n65 = Concatenate Strings("Bi-Dir B-scan(x): " ("string"), "Enable") -> (w138:string)
              n66 = Bundle(w138, "double precision float"=1.0) -> (w137:cluster{string, "double precision float":dbl})  [unwired: 1 in]
              n67 = Write to Binary File(file (use dialog)=w141, data=w137, 9:w140) -> ()  [unwired: 2 in, 4 out]
            }
            frame #9 {
              n68 = Concatenate Strings("Dual Wavelength:" ("string"), "Disable") -> (w144:string)
              n69 = Bundle(w144, 0.0) -> (w145:cluster{string, dbl})  [unwired: 1 in]
              n70 = Write to Binary File(file (use dialog)=w148, data=w145, 9:w147) -> ()  [unwired: 2 in, 4 out]
            }
            frame #10 {
              n71 = local read "Laser Rep Rate"() -> (w149:u32)
              n72 = To Double Precision Float(number=w149) -> (double precision float=w152:dbl)
              n73 = Number To Fractional String(number=w149, precision (6)=i16 2) -> (F-format string=w156:string)  [unwired: 2 in]
              n74 = Concatenate Strings("Laser Rep Rate(Hz): " ("string"), w156) -> (w150:string)
              n75 = Bundle(w150, w152) -> (w151:cluster{string, dbl})  [unwired: 1 in]
              n76 = Write to Binary File(file (use dialog)=w154, data=w151, 9:w153) -> ()  [unwired: 2 in, 4 out]
            }
            frame #11 {
              w158 = 0.0 ("number")
              n77 = Number To Fractional String(number=w158, precision (6)=i16 8) -> (F-format string=w165:string)  [unwired: 2 in]
              n78 = Concatenate Strings("Laser time interval: " ("string"), w165) -> (w159:string)
              n79 = To Double Precision Float(number=w158) -> (double precision float=w161:dbl)
              n80 = Bundle(w159, w161) -> (w160:cluster{string, dbl})  [unwired: 1 in]
              n81 = Write to Binary File(file (use dialog)=w163, data=w160, 9:w162) -> ()  [unwired: 2 in, 4 out]
            }
            frame #12 {
              n82 = local read "Pt per A-line"() -> (w167:i32)
              n83 = To Double Precision Float(number=w167) -> (double precision float=w170:dbl)
              n84 = Number To Fractional String(number=w167, precision (6)=i16 2) -> (F-format string=w174:string)  [unwired: 2 in]
              n85 = Concatenate Strings("Pt per Aline: " ("string"), w174) -> (w168:string)
              n86 = Bundle(w168, w170) -> (w169:cluster{string, dbl})  [unwired: 1 in]
              n87 = Write to Binary File(file (use dialog)=w171, data=w169, 9:w172) -> ()  [unwired: 2 in, 4 out]
            }
            frame #13 {
              n88 = local read "Mode"() -> (w176:enum32{"Continuous", "Discrete"})
              n89 = Equal?(x=w176, y=enum32{"Continuous", "Discrete"}."Continuous" ("Elevational Mode")) -> (x = y?=w181:bool)
              n90 = Select(t="Continuous", s=w181, f="Discrete") -> (s? t:f=w185:string)
              n91 = Concatenate Strings("Elevational (y) Scan Mode: " ("string"), w185) -> (w177:string)
              n92 = To Double Precision Float(number=w176) -> (double precision float=w179:dbl)
              n93 = Bundle(w177, w179) -> (w178:cluster{string, dbl})  [unwired: 1 in]
              n94 = Write to Binary File(file (use dialog)=w184, data=w178, 9:w183) -> ()  [unwired: 2 in, 4 out]
            }
            frame #14 {
              n95 = local read "Ele_Ini_Dir"() -> (w189:bool)
              n96 = Select(t="Towards Motor", s=w189, f="Away Motor") -> (s? t:f=w195:string)
              n97 = Boolean To (0,1)(Boolean=w189) -> (0, 1=w188:i16)
              n98 = Concatenate Strings("Y Direction:" ("string"), w195) -> (w191:string)
              n99 = To Double Precision Float(number=w188) -> (double precision float=w192:dbl)
              n100 = Bundle(w191, w192) -> (w190:cluster{string, dbl})  [unwired: 1 in]
              n101 = Write to Binary File(file (use dialog)=w194, data=w190, 9:w193) -> ()  [unwired: 2 in, 4 out]
            }
            frame #15 {
              n102 = Build Array("CH_A", "CH_B", "CH_A_B") -> (w204:string[])
              n103 = local read "Channel"() -> (w199:T1)
              n104 = Index Array(array=w204, index=w199) -> (element=w203:string)
              n105 = To Double Precision Float(number=w199) -> (double precision float=w202:dbl)
              n106 = Concatenate Strings("Chan: " ("string"), w203) -> (w201:string)
              n107 = Bundle(w201, w202) -> (w200:cluster{string, dbl})  [unwired: 1 in]
              n108 = Write to Binary File(file (use dialog)=w209, data=w200, 9:w208) -> ()  [unwired: 2 in, 4 out]
            }
            frame #16 {
              n109 = To Double Precision Float(number=0.0) -> (double precision float=w212:dbl)
              n110 = Bundle("/*END*/", w212) -> (w213:cluster{string, dbl})  [unwired: 1 in]
              n111 = Write to Binary File(file (use dialog)=w215, data=w213, 9:w216) -> ()  [unwired: 2 in, 4 out]
            }
          }
        }
        frame Enabled {
        }
      }
      n112 = call <vilib>:"Signal Generator by Duration.vi"("signal type"="signal type", "reset phase"=TRUE, "# of samples"=w14, "frequency"=1.0, "amplitude"="Range (V)", "dc offset"="Offset (V)", "phase in"="Phase0(deg)") -> ("signal"=w49:dbl[])  [unwired: 5 in, 3 out]
      n113 = Scale By Power Of 2(n=w18, x=u8 1 ("bit")) -> (x*2^n=w33:u8)
      n114 = Array Size(array=w21) -> (size(s)=w34:i32)
      n115 = Obtain Queue(name (unnamed)="DAQ1", element data type=u16[] [] ("Buffer")) -> (queue out=→"DataQueue":refnum<queue>)  [unwired: 3 in, 2 out]
      n116 = local read "yEn"() -> (w28:bool)
      n117 = Multiply(x=w49, y=204.8 ("frequency")) -> (x*y=w61:dbl[])
      n118 = To Word Integer(number=w61) -> (16bit integer=→"Galvo Mirror Traj":i16[])
      n119 = Quotient & Remainder(x=40000000, y="Laser Rep Rate") -> (floor(x/y)=w10:u32)  [unwired: 1 out]
      n120 = local read "GMnum"() -> (w4:i16)
      n121 = Quotient & Remainder(x="Laser Rep Rate", y=w4) -> (floor(x/y)=w3:u32)  [unwired: 1 out]
      n122 = local read "dy"() -> (w2:i32)
      n123 = Multiply(x=w10, y=w4) -> (x*y=w9:u32)
      n124 = Multiply(x=w3, y=w2) -> (x*y=→"Motorfreq_hz= Laserfre*dy/GMnum":u32)
      n125 = local write "Laserupdateus"(w10) -> ()
      n126 = local read "DO_rate_tick"() -> (w8:u32)
      n127 = Quotient & Remainder(x=w9, y=w8) -> (floor(x/y)=w7:u32)  [unwired: 1 out]
      n128 = Multiply(x=w42, y=w7) -> (x*y=w31:dbl)
      n129 = call "generatepulse.vi"("en"=w28, "samples"=w31, "bit"=u8 1, "dir"=FALSE, "xn"=w30) -> ("pulsetrain"=w27:u8[])  [unwired: 6 in]
      n130 = Subtract(x=w31, y=w34) -> (x-y=w39:dbl)
      n131 = Initialize Array(w33, w39) -> (w35:u8[])
      n132 = Insert Into Array(array=w21, index=0, new element=w35) -> (w36:u8[])
      n133 = Add(x=w27, y=w36) -> (x+y=w37:u8[])
      n134 = Exclusive Or(1:u8 2 ("bit"), 2:w37) -> (0:w38:u8[])
      n135 = local write "Pulses"(w37) -> ()
      n136 = local write "Pulsesb"(w38) -> ()
      n137 = local write "Stop_dispaly"(FALSE ("Stop_dispaly")) -> ()
      n138 = local write "Timesperdx"(w7) -> ()
      "B-scan saved" <- 0 ("saved bscan")
    }
    frame #1 {
      (unwired) i16 32000 ("pls_V")
      n139 = local read "DAQ Trig #"() -> (w274:i32)
      n140 = xnode "Open FPGA VI Reference"("resource name"=T6 "rio://172.22.11.2/RIO0") -> ("FPGA VI Reference Out"=w280:refnum<k20>, "error out"=w281:errorcluster)  [unwired: 1 in]
      n141 = xnode "Invoke Method"("FPGA VI Reference In"=w280, "error in"=w281) -> ("FPGA VI Reference Out"=w282:refnum<k20>, "error out"=w283:errorcluster)
      n142 = Multiply(x=w274, y=2) -> (x*y=w273:i32)
      n143 = xnode "Invoke Method"("FPGA VI Reference In"=w282, "error in"=w283, "Requested Depth"=w273) -> ("FPGA VI Reference Out"=w234:refnum<k20>, "error out"=w233:errorcluster)  [unwired: 1 out]
      n144 = local read "Galvo Mirror Traj"() -> (w264:i16[])
      n145 = call "TrigGenEdgewave.vi"() -> ("Digital Waveform Graph"=→"Trigger pulse graph 2":digitalwaveform, "delays"=w241:u32[])  [unwired: 10 in]
      n146 = local read "GMnum"() -> (w229:i16)
      n147 = local read "yn"() -> (w227:i32)
      n148 = xnode "Invoke Method"("FPGA VI Reference In"=w234, "error in"=w233, "Data"=w264) -> ("FPGA VI Reference Out"=w271:refnum<k20>, "error out"=w284:errorcluster)  [unwired: 1 in, 1 out]
      n149 = local read "dy"() -> (w226:i32)
      n150 = local read "DAQ Trig #"() -> (w244:i32)
      n151 = Multiply(x=w227, y=w226) -> (x*y=w225:i32)
      n152 = local read "dx"() -> (w219:i32)
      n153 = Quotient & Remainder(x=w229, y=w226) -> (floor(x/y)=w228:i32)  [unwired: 1 out]
      n154 = Multiply(x=w227, y=w229) -> (x*y=w230:i32)
      n155 = local read "Laserupdateus"() -> (w235:u32)
      n156 = Multiply(x=w219, y="Zdiv") -> (x*y=w220:i32)
      n157 = local read "xn"() -> (w240:i32)
      n158 = Not(x="Ele_Ini_Dir") -> (.not. x?=w265:bool)
      n159 = Subtract(x=w225, y=w220) -> (x-y=w232:i32)
      n160 = Multiply(x=w230, y=w240) -> (x*y=w237:i32)
      n161 = local read "zdir"() -> (w231:bool)
      n162 = xnode "Read/Write Control"("FPGA VI Reference In"=w271, "error in"=w284, "FIFO_Timeout"=-1, "stop 2"=FALSE ("stop"), "Ele_Ini_Dir"=w265, "start_scan"=FALSE, "VC_pt_in_fifo"=w244, "Zdir"=w231, "Laserupdateus"=w235, "LON"=TRUE, "Zmotorbackspeedticks"=u32 40000, "VC_pt_nm"=w244, "LsrCtrl"=40, "delays"=w241, "LaserNum"=w237, "Xn-dz"=w232, "Laser/xn/dx"=w228, "Stepm_pt_nm"=w230, "Zdiv"="Zdiv") -> ("FPGA VI Reference Out"=w278:refnum<k20>, "error out"=w275:errorcluster)
      n163 = local write "Laser fired"(w237) -> ()
      n164 = case shown="True" "Big_data" {
        frame False {
        }
        frame True {
          n165 = while {
            stop <- w285 stop-if-true
            n166 = local read "DataQueue"() -> (w292:refnum<queue>)
            n167 = local read "Stop_dispaly"() -> (w286:bool)
            n168 = Get Queue Status(queue=w292) -> (queue out=w290:refnum<queue>, # elements in queue=w289:i32)  [unwired: 2 in, 6 out]
            n169 = Wait Until Next ms Multiple(millisecond multiple="save_rate") -> ()  [unwired: 1 out]
            n170 = Equal To 0?(x=w289) -> (x = 0?=w287:bool)
            n171 = And(x=w287, y=w286) -> (x .and. y?=w285:bool)
            n172 = Greater Than 0?(x=w289) -> (x > 0?=w291:bool)
            n173 = case shown="True" w291 {
              tunnel: w290 -> [_ w310]
              frame False {
                n174 = Wait Until Next ms Multiple(millisecond multiple=u32 5) -> ()  [unwired: 1 out]
              }
              frame True {
                # "two channel is 2\none channel is 1"
                n175 = Dequeue Element(queue=w310) -> (element=w299:u16[])  [unwired: 2 in, 3 out]
                n176 = local read "catbscan"() -> (w307:i16)
                n177 = local read "Alines"() -> (w308:i32)
                n178 = local read "Pt per A-line"() -> (w303:i32)
                n179 = local read "catbscan"() -> (w298:i16)
                n180 = Multiply(x=w307, y=w308) -> (x*y=w296:i32)
                n181 = local read "B-scan saved"() -> (w304:i32)
                n182 = Multiply(x=w296, y=1) -> (x*y=w294:i32)
                n183 = Reshape Array(w299, w294, w303) -> (w306:u16[][])
                n184 = case shown="True" "A/B-line show" {
                  tunnel: w299 -> [_ _]
                  tunnel: w306 -> [_ w312]
                  frame False {
                  }
                  frame True {
                    # "every 20 buffer show once\nand then show the 21th buffer"
                    n185 = local read "B-scan saved"() -> (w316:i32)
                    n186 = local read "catbscan"() -> (w317:i16)
                    n187 = local read "catbscan"() -> (w311:i16)
                    n188 = Multiply(x=w317, y=1) -> (x*y=w319:i32)
                    n189 = Quotient & Remainder(x=w316, y=w319) -> (x-y*floor(x/y)=w314:i32)  [unwired: 1 out]
                    n190 = Equal To 0?(x=w314) -> (x = 0?=w315:bool)
                    n191 = Equal?(x=w314, y=w311) -> (x = y?=w313:bool)
                    n192 = case shown="True" w315 {
                      tunnel: w312 -> [_ w321]
                      frame False {
                      }
                      frame True {
                        "B-Scan" <- w321
                        "Waveform Graph" <- w321
                      }
                    }
                    n193 = case shown="True" w313 {
                      tunnel: w312 -> [_ w320]
                      frame False {
                      }
                      frame True {
                        "B-Scan 2" <- w320
                      }
                    }
                  }
                }
                n194 = Add(x=w304, y=w298) -> (x+y=w305:i32)
                n195 = local write "B-scan saved"(w305) -> ()
                n196 = case shown="True" "Calc MAP" {
                  tunnel: w296 -> [_ w329]
                  tunnel: w304 -> [_ w328]
                  tunnel: w306 -> [_ w327]
                  tunnel: [u16[] [] w325] -> w300
                  frame False {
                  }
                  frame True {
                    n197 = case shown="False" "Dual Wave" {
                      tunnel: w329 -> [w334 w347]
                      tunnel: w327 -> [w333 w346]
                      tunnel: [w331 w345] -> w325
                      tunnel: [w330 w345] -> w324
                      frame True {
                        n198 = for {
                          N: w334 -> [_]
                          tunnel: w333 -> [w341] mode=indexing
                          tunnel: [w344] -> w330 mode=indexing
                          tunnel: [w337] -> w332 mode=indexing
                          n199 = Split 1D Array(array=w341, index="Split") -> (first subarray=w335:u16[], second subarray=w336:u16[])
                          n200 = Array Max & Min(array=w336) -> (max value=w343:u16, min value=w342:u16)  [unwired: 2 out]
                          n201 = Array Max & Min(array=w335) -> (max value=w339:u16, min value=w338:u16)  [unwired: 2 out]
                          n202 = Subtract(x=w343, y=w342) -> (x-y=w344:u16)
                          n203 = Subtract(x=w339, y=w338) -> (x-y=w337:u16)
                        }
                        n204 = Interleave 1D Arrays(w330, w332) -> (w331:u16[])
                      }
                      frame False {
                        n205 = for {
                          N: w347 -> [_]
                          tunnel: w346 -> [w348] mode=indexing
                          tunnel: [w351] -> w345 mode=indexing
                          n206 = Array Max & Min(array=w348) -> (max value=w350:u16, min value=w349:u16)  [unwired: 2 out]
                          n207 = Subtract(x=w350, y=w349) -> (x-y=w351:u16)
                        }
                      }
                    }
                    n208 = case shown="True" "showmap" {
                      selector: "showmap" -> [_ w352]
                      tunnel: w328 -> [_ w368]
                      tunnel: w324 -> [_ w355]
                      frame False {
                      }
                      frame True {
                        n209 = local read "B-scan #"() -> (w361:u32)
                        n210 = Subtract(x=w361, y=1) -> (x-y=w365:u32)
                        n211 = local read "Alines"() -> (w359:i32)
                        n212 = local read "catbscan"() -> (w360:i16)
                        n213 = Reshape Array(w355, w360, w359) -> (w356:u16[][])
                        n214 = Quotient & Remainder(x=w368, y=w361) -> (x-y*floor(x/y)=w364:u32, floor(x/y)=w367:u32)
                        n215 = Subtract(x=w365, y=w364) -> (x-y=w363:u32)
                        n216 = And(x=w367, y=1) -> (x .and. y?=w362:u32)
                        n217 = Transpose 2D Array(2D array=w356) -> (transposed array=w358:u16[][])
                        n218 = Greater Than 0?(x=w362) -> (x > 0?=w354:bool)
                        n219 = And(x=w354, y=w352) -> (x .and. y?=w353:bool)
                        n220 = case shown="True" w353 {
                          tunnel: w358 -> [w369 w380]
                          tunnel: w364 -> [_ w379]
                          tunnel: w363 -> [w370 _]
                          frame False {
                            n221 = disable-structure shown="Disabled" {
                              disable-tunnel: w370 -> [w375 _]
                              disable-tunnel: w369 -> [w374 _]
                              frame Disabled {
                                n222 = local read "MAP"() -> (w372:u16[][])
                                n223 = Replace Array Subset(array=w372, new element=w374, index (row)=0 ("disabled index (row)"), index (col)=w375) -> (w373:u16[][])
                                n224 = local write "MAP"(w373) -> ()
                              }
                              frame Enabled {
                              }
                            }
                          }
                          frame True {
                            n225 = local read "MAP"() -> (w377:u16[][])
                            n226 = Replace Array Subset(array=w377, new element=w380, index (row)=0 ("disabled index (row)"), index (col)=w379) -> (w378:u16[][])
                            n227 = local write "MAP"(w378) -> ()
                          }
                        }
                      }
                    }
                  }
                }
                n228 = Select(t=w300, s="Savemap", f=w299) -> (s? t:f=→"s? t:f":u16[])
              }
            }
          }
        }
      }
      n229 = flat-sequence {
        tunnel: w278 -> [w385]
        tunnel: w275 -> [w382]
        tunnel: [w384] -> w268
        tunnel: [w383] -> w267
        tunnel: w268 -> [w404]
        tunnel: w267 -> [w403]
        tunnel: [w404] -> w263
        tunnel: [w403] -> w261
        tunnel: [w396] -> w255
        tunnel: [w389] -> w252
        tunnel: [w395] -> w249
        tunnel: ["Pt per A-line"] -> w246
        tunnel: w263 -> [w413]
        tunnel: [w413] -> w262
        tunnel: w261 -> [w412]
        tunnel: [w412] -> w260
        tunnel: [w410] -> w256
        tunnel: w255 -> [w410]
        tunnel: [w409] -> w253
        tunnel: w252 -> [w409]
        tunnel: [w407] -> w250
        tunnel: w249 -> [w406]
        tunnel: [w408] -> w247
        tunnel: w246 -> [w408]
        tunnel: w262 -> [w422]
        tunnel: w260 -> [w420]
        tunnel: [w421] -> w259
        tunnel: [w419] -> w258
        tunnel: [w417] -> w257
        tunnel: w256 -> [w417]
        tunnel: [w416] -> w254
        tunnel: w253 -> [w416]
        tunnel: [w415] -> w251
        tunnel: w250 -> [w415]
        tunnel: [w414] -> w248
        tunnel: w247 -> [w414]
        tunnel: w259 -> [w432]
        tunnel: w258 -> [w431]
        tunnel: w257 -> [w430]
        tunnel: w254 -> [w428]
        tunnel: w251 -> [w426]
        tunnel: w248 -> [w425]
        tunnel: [w432] -> w223
        tunnel: [w431] -> w222
        tunnel: [w423] -> w221
        tunnel: [w473] -> w236
        tunnel: [w474] -> w238
        tunnel: [w475] -> w239
        tunnel: w223 -> [w475]
        tunnel: w222 -> [w474]
        tunnel: w221 -> [w473]
        frame #0 {
          n230 = xnode "Invoke Method"("FPGA VI Reference In"=w385, "error in"=w382) -> ("FPGA VI Reference Out"=w384:refnum<k20>, "error out"=w383:errorcluster)  [unwired: 1 in]
          n231 = Wait Until Next ms Multiple(millisecond multiple=u32 2) -> ()  [unwired: 1 out]
        }
        frame #1 {
          # "channel equals A+B, here set 2\nequals A, SET 1"
          # "you may set total records\nhere, if one day you need to \nget too much data,revise here to infinity"
          n232 = local read "DAQ Trig #"() -> (w398:i32)
          "Alines" <- w398
          n233 = local read "Laser fired"() -> (w387:i32)
          n234 = local read "catbscan"() -> (w397:i16)
          n235 = local read "B-scan #"() -> (w399:u32)
          n236 = Multiply(x=w387, y=1.0) -> (x*y=w386:dbl)
          n237 = Multiply(x=w398, y=w397) -> (x*y=w395:i32)
          n238 = Initialize Array(u16 0 ("element"), w398, w399) -> (→"MAP":u16[][])
          n239 = Multiply(x="Pt per A-line", y=w398) -> (x*y=→"Ch1 Pt":i32)
          n240 = call "ATS9350_NPT_Scan.vi"("Records per Buffer"=w395, "Pt per A-line"="Pt per A-line", "Total records number"=w386, "Numeric"="Trig. Delay (us)", "Range"="ChA_Range") -> ("Device ID"=w396:u64)  [unwired: 10 in]
          n241 = Multiply(x="Pt per A-line", y=w395) -> (x*y=w391:i32)
          n242 = Multiply(x=w391, y=1) -> (x*y=w389:i32)
        }
        frame #2 {
          # "for two channel, displayed should be twice the records per buffer"
          # "buffer size"
          n243 = Multiply(x=w406, y=1) -> (x*y=w407:i32)
          n244 = Wait Until Next ms Multiple(millisecond multiple=u32 200) -> ()  [unwired: 1 out]
        }
        frame #3 {
          n245 = xnode "Read/Write Control"("FPGA VI Reference In"=w422, "error in"=w420, "start_scan"=TRUE) -> ("FPGA VI Reference Out"=w421:refnum<k20>, "error out"=w419:errorcluster)
        }
        frame #4 {
          n246 = Initialize Array(u16 0 ("element"), w428) -> (w427:u16[])
          n247 = while {
            tunnel: w427 -> [w447]
            shift-right: [w435] -> w424
            shift-left: w430 -> [w448]
            tunnel: w426 -> [w445]
            tunnel: w425 -> [w444]
            tunnel: [w433] -> w423
            stop <- w433 stop-if-true
            # "records per buffer"
            # "Aline points num"
            # "Clear WaitTimeout"
            # "Display buffer if valid:\n - Code 512: ApiSuccess\n - Code 589: ApiTransferComplete"
            # "Clear Transf. Complete"
            n248 = call "AlazarWaitNextAsyncBufferCompleteU16.vi"("Timeout (ms)"=u32 100, "Buffer"=w447, "Handle"=w448) -> ("error out"=w438:errorcluster, "Return Code"=w437:u32, "Buffer"=w434:u16[], "Handle"=w436:u64)  [unwired: 1 in]
            n249 = case shown="512, 589" w437 {
              tunnel: w434 -> [_ w464]
              tunnel: w445 -> [_ w470]
              tunnel: w444 -> [_ w469]
              frame Default {
              }
              frame 512, 589 {
                n250 = local read "file_ref"() -> (w468:refnum<file>)
                n251 = local read "DataQueue"() -> (w463:refnum<queue>)
                n252 = Reshape Array(w464, w470, w469) -> (→"Graph":u16[][])
                n253 = Write to Binary File(file (use dialog)=w468, data=w464, 5:FALSE ("prepend array or string size? (T)"), 9:T5."native, host order" ("byte order (0:big-endian, network order)")) -> (error out=w467:errorcluster)  [unwired: 1 in, 3 out]
                n254 = Enqueue Element(queue=w463, element=w464) -> ()  [unwired: 2 in, 3 out]
                n255 = call <vilib>:"Simple Error Handler.vi"("error in (no error)"=w467) -> ()  [unwired: 4 in, 5 out]
              }
            }
            n256 = case shown="579" w437 {
              selector: w437 -> [w457 w459]
              tunnel: w438 -> [w456 w462]
              tunnel: [w456 w461] -> w443
              tunnel: [w458 w460] -> w442
              tunnel: w436 -> [w458 w460]
              tunnel: [w457 w459] -> w441
              frame 0, Default {
              }
              frame 579 {
                n257 = call <vilib>:"Clear Errors.vi"("error in (no error)"=w462) -> ("error out"=w461:errorcluster)  [unwired: 5 in, 1 out]
              }
            }
            n258 = Unbundle By Name(w443) -> ("status"=w439:bool)
            n259 = case shown="0, Default" w441 {
              selector: w441 -> [w450 w452]
              tunnel: w443 -> [w449 w455]
              tunnel: [w449 w454] -> _
              tunnel: [w451 w453] -> w435
              tunnel: w442 -> [w451 w453]
              tunnel: [w450 w452] -> _
              frame 0, Default {
              }
              frame 589 {
                n260 = call <vilib>:"Clear Errors.vi"("error in (no error)"=w455) -> ("error out"=w454:errorcluster)  [unwired: 5 in, 1 out]
              }
            }
            n261 = Or(x="stop 2", y=w439) -> (x .or. y?=w433:bool)
          }
          n262 = call "AlazarAbortAsyncRead.vi"("Handle"=w424) -> ()  [unwired: 1 in, 3 out]
        }
        frame #5 {
          # "Wait motor back, \nthen close fpga"
          n263 = Wait (ms)(milliseconds to wait=u32 5000) -> ()  [unwired: 1 out]
        }
      }
      n264 = xnode "Close FPGA VI Reference"("FPGA VI Reference In"=w239, "error in"=w238) -> ("error out"=w277:errorcluster)
      n265 = local write "Stop_dispaly"(w236) -> ()
      n266 = call <vilib>:"Simple Error Handler.vi"("error in (no error)"=w277) -> ()  [unwired: 4 in, 5 out]
    }
    frame #2 {
      n267 = local read "DataQueue"() -> (w477:refnum<queue>)
      n268 = local read "file_ref"() -> (w476:refnum<file>)
      n269 = Release Queue(queue=w477) -> ()  [unwired: 2 in, 3 out]
      n270 = Close File(refnum=w476) -> ()  [unwired: 1 in, 2 out]
    }
  }
